vi "CRYAPI Pic PreDOCKING.vi"(8 "nDWinID":i32, 9 "nSWinID":i32, 11 "sAction":string) -> (0 "bResult":bool=TRUE)   [LabVIEW 2013]
uses:
  CRYMain Sub Window Global.vi
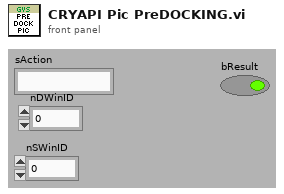
[diagram p1: front panel]
types:
  T1 = typedef "LVRectTypeDef.ctl" = cluster{"Left":i16, "Top":i16, "Right":i16, "Bottom":i16}
  T2 = cluster{"nType":i32, "nParent":i32, "pVIW":refnum<vi>, "pSPW":refnum<vi>, "nTypeF":i32, "pVIF":refnum<vi>, "pSPF":refnum<vi>, "nIDSpliter":i32, "nProperty":i32, "Bound":T1, "nID":i32, "nData":i32, "sData":string, "pWVI":refnum<vi>, "sTitle":string, "cPages":cluster{"nPage":i32, "sTitle":string, "sIcon":string, "pVI":refnum<vi>, "nID":i32}[], "pTab":refnum<vi>, "nIDPages":i32[], "pSPT":refnum<vi>, "sTemp":string, "nDockID":i32, "nDockLR":i32, "sIcon":string}
  T3 = typedef "LVPointTypeDef.ctl" = cluster{"Horizontal":i16, "Vertical":i16}
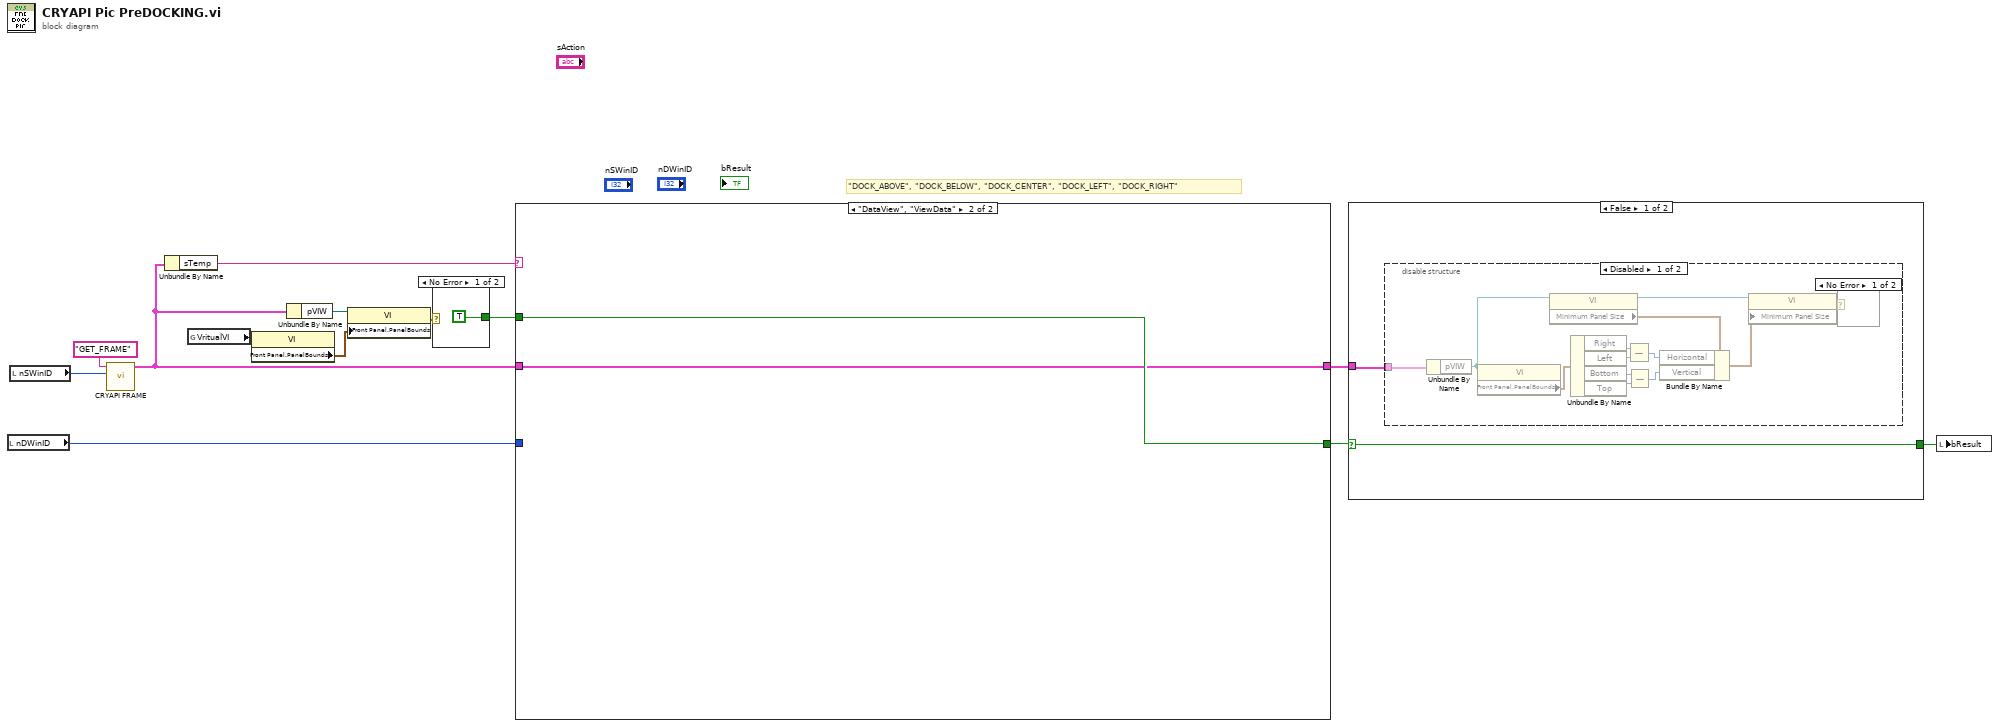
[diagram p0: block diagram]
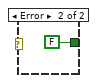
[diagram p5: hidden frame]
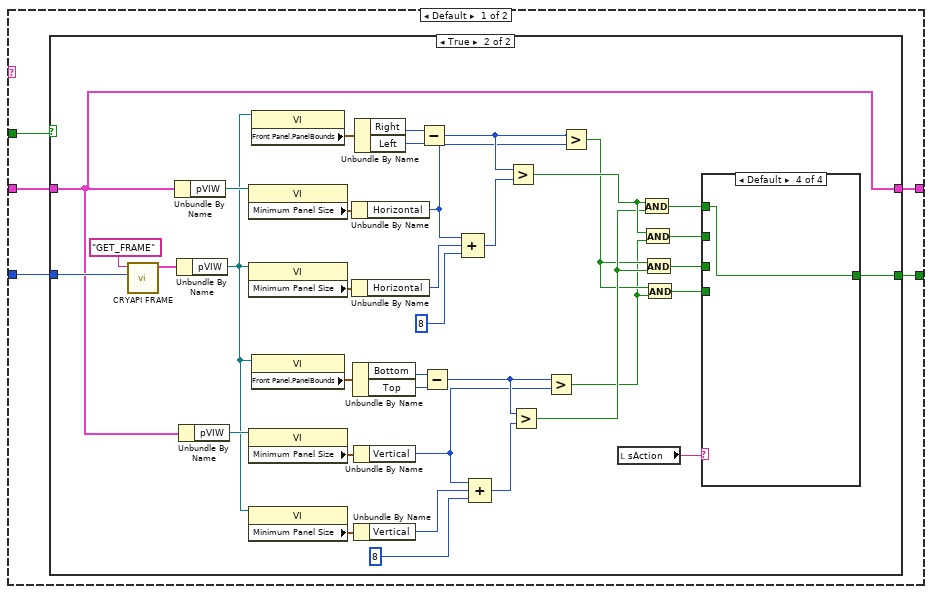
[diagram p6: hidden frame]
diagram:
  # "\"DOCK_ABOVE\", \"DOCK_BELOW\", \"DOCK_CENTER\", \"DOCK_LEFT\", \"DOCK_RIGHT\""
  n1 = local read "nDWinID"() -> (w11:i32)
  n2 = local read "nSWinID"() -> (w12:i32)
  n3 = call "CRYAPI FRAME.vi"("nData"=w12, "sAction"="GET_FRAME") -> ("tFrame_Out"=w4:T2)  [unwired: 4 in, 5 out]
  n4 = Unbundle By Name(w4) -> ("sTemp"=w10:string)
  n5 = global read "CRYMain Sub Window Global.vi" "VritualVI"() -> (w8:refnum<vi>)
  n6 = property class="VI"(reference=w8) -> ("Front Panel.PanelBounds"=w6:T1)  [unwired: 1 in, 2 out]
  n7 = Unbundle By Name(w4) -> ("pVIW"=w7:refnum<vi>)
  n8 = property class="VI"(reference=w7, "Front Panel.PanelBounds"=w6) -> (error out=w9:errorcluster)  [unwired: 1 in, 1 out]
  n9 = case shown="No Error" w9 {
    tunnel: [TRUE FALSE] -> w5
    frame No Error {
    }
    frame Error {
    }
  }
  n10 = case shown="\"DataView\", \"ViewData\"" w10 {
    tunnel: w4 -> [w19 w64]
    tunnel: w11 -> [w20 _]
    tunnel: [w17 w65] -> w3
    tunnel: w5 -> [w18 w65]
    tunnel: [w16 w64] -> w1
    frame Default {
      n11 = case shown="True" w18 {
        selector: w18 -> [w22 _]
        tunnel: w20 -> [_ w39]
        tunnel: w19 -> [w21 w23]
        tunnel: [w22 w24] -> w17
        tunnel: [w21 w23] -> w16
        frame False {
        }
        frame True {
          n12 = call "CRYAPI FRAME.vi"("nData"=w39, "sAction"="GET_FRAME") -> ("tFrame_Out"=w44:T2)  [unwired: 4 in, 5 out]
          n13 = Unbundle By Name(w23) -> ("pVIW"=w49:refnum<vi>)
          n14 = Unbundle By Name(w44) -> ("pVIW"=w25:refnum<vi>)
          n15 = Unbundle By Name(w23) -> ("pVIW"=w52:refnum<vi>)
          n16 = property class="VI"(reference=w49) -> ("Minimum Panel Size"=w50:T3)  [unwired: 1 in, 2 out]
          n17 = property class="VI"(reference=w25) -> ("Minimum Panel Size"=w45:T3)  [unwired: 1 in, 2 out]
          n18 = property class="VI"(reference=w52) -> ("Minimum Panel Size"=w51:T3)  [unwired: 1 in, 2 out]
          n19 = property class="VI"(reference=w25) -> ("Minimum Panel Size"=w56:T3)  [unwired: 1 in, 2 out]
          n20 = property class="VI"(reference=w25) -> ("Front Panel.PanelBounds"=w48:T1)  [unwired: 1 in, 2 out]
          n21 = property class="VI"(reference=w25) -> ("Front Panel.PanelBounds"=w53:T1)  [unwired: 1 in, 2 out]
          n22 = Unbundle By Name(w50) -> ("Horizontal"=w30:i16)
          n23 = Unbundle By Name(w45) -> ("Horizontal"=w42:i16)
          n24 = Unbundle By Name(w53) -> ("Bottom"=w55:i16, "Top"=w54:i16)
          n25 = Unbundle By Name(w51) -> ("Vertical"=w36:i16)
          n26 = Unbundle By Name(w56) -> ("Vertical"=w57:i16)
          n27 = Unbundle By Name(w48) -> ("Right"=w46:i16, "Left"=w47:i16)
          n28 = Subtract(x=w46, y=w47) -> (x-y=w31:i16)
          n29 = Subtract(x=w55, y=w54) -> (x-y=w37:i16)
          n30 = Compound Arithmetic op=ADD(w30, w42, i16 8 ("value")) -> (w40:i16)
          n31 = Compound Arithmetic op=ADD(w36, w57, i16 8 ("value")) -> (w59:i16)
          n32 = Greater?(x=w31, y=w40) -> (0:w34:bool)
          n33 = Greater?(x=w37, y=w59) -> (0:w32:bool)
          n34 = Greater?(x=w37, y=w36) -> (0:w27:bool)
          n35 = Greater?(x=w31, y=w30) -> (0:w28:bool)
          n36 = local read "sAction"() -> (w38:string)
          n37 = And(x=w34, y=w32) -> (x .and. y?=w35:bool)
          n38 = And(x=w34, y=w27) -> (x .and. y?=w33:bool)
          n39 = And(x=w28, y=w32) -> (x .and. y?=w29:bool)
          n40 = And(x=w28, y=w27) -> (x .and. y?=w26:bool)
          n41 = case shown="Default" w38 {
            tunnel: w35 -> [_ _ _ w63]
            tunnel: [w60 w61 w62 w63] -> w24
            tunnel: w33 -> [w60 _ _ _]
            tunnel: w29 -> [_ w61 _ _]
            tunnel: w26 -> [_ _ w62 _]
            frame "DOCK_LEFT", "DOCK_RIGHT" {
            }
            frame "DOCK_ABOVE", "DOCK_BELOW" {
            }
            frame "DOCK_CENTER" {
            }
            frame Default {
            }
          }
        }
      }
    }
    frame "DataView", "ViewData" {
    }
  }
  n42 = case shown="False" w3 {
    selector: w3 -> [w67 w81]
    tunnel: [w67 w81] -> w2
    tunnel: w1 -> [w66 _]
    frame False {
      n43 = disable-structure shown="Disabled" {
        disable-tunnel: w66 -> [w80 _]
        frame Disabled {
          n44 = Unbundle By Name(w80) -> ("pVIW"=w74:refnum<vi>)
          n45 = property class="VI"(reference=w74) -> ("Front Panel.PanelBounds"=w79:T1)  [unwired: 1 in, 2 out]
          n46 = property class="VI"(reference=w74) -> (reference out=w70:refnum<vi>, "Minimum Panel Size"=w73:T3)  [unwired: 1 in, 1 out]
          n47 = Unbundle By Name(w79) -> ("Right"=w77:i16, "Left"=w78:i16, "Bottom"=w76:i16, "Top"=w75:i16)
          n48 = Subtract(x=w77, y=w78) -> (x-y=w72:i16)
          n49 = Subtract(x=w76, y=w75) -> (x-y=w71:i16)
          n50 = Bundle By Name(cluster=w73, "Horizontal"=w72, "Vertical"=w71) -> (w69:T3)
          n51 = property class="VI"(reference=w70, "Minimum Panel Size"=w69) -> (error out=w68:errorcluster)  [unwired: 1 in, 1 out]
          n52 = case shown="No Error" w68 {
            frame No Error {
            }
            frame Error {
            }
          }
        }
        frame Enabled {
        }
      }
    }
    frame True {
    }
  }
  n53 = local write "bResult"(w2) -> ()
